vi "Estimate2DAffineVariableScale.vi"(8 "error in":errorcluster, 10 "To":map{i32, T1}(c390), 11 "From":map{i32, T1}(c390)) -> (0 "error out":errorcluster, 1 "c":dbl, 2 "T":T1, 3 "R":T2)   [LabVIEW 2020, in "ar.lvlib"]
doc: "Estimate an Affine Transformation between sets of points."
uses:
  ar.lvlib
  common/Image Point (Float).ctl
  <vilib>/Analysis/Matrix/Datatypes/RealMatrix.ctl
  1dd33249-2402-4cc2-9784-1d2efc93c5c7.vi
  SubtractMeanFromPoints.vi
  CovarianceofPointSetsA&B.vi
  DecomposeCovarianceOfPointSetsA&B.vi
  <vilib>/Analysis/baseanly.llb/A x Vector.vi
  <vilib>/Analysis/baseanly.llb/Mean.vi
  <vilib>/Analysis/baseanly.llb/Mean (DBL).vi
  <vilib>/Analysis/baseanly.llb/A x B.vi
  <vilib>/Analysis/baseanly.llb/Real A x B.vi
  <vilib>/Analysis/baseanly.llb/Determinant.vi
  <vilib>/Analysis/baseanly.llb/Real Determinant.vi
  SVDForPointSetCovarainces.vi
  <vilib>/Analysis/_algsub.llb/Matrix Rank.vi
  <vilib>/Analysis/_algsub.llb/Real Matrix Rank.vi
  <vilib>/Analysis/_algsub.llb/Trace.vi
  <vilib>/Analysis/_algsub.llb/Real Matrix Trace.vi
  <vilib>/Utility/error.llb/Error Cluster From Error Code.vi
  <vilib>/Analysis/Matrix/Numeric/Conversions/Array To Matrix - RA2.vi
  <vilib>/Analysis/7linalg.llb/SVD Decomposition.vi
  <vilib>/Analysis/7linalg.llb/Real SVD Decomposition.vi
  <vilib>/Analysis/7linalg.llb/Create Special Matrix.vi
  <vilib>/Analysis/7linalg.llb/Create Special Real Matrix.vi
  <vilib>/Analysis/Matrix/Numeric/Multiply/Multiply - RM,R.vi
  common/common.lvlib
  <vilib>/Analysis/Matrix/NI_Matrix.lvlib
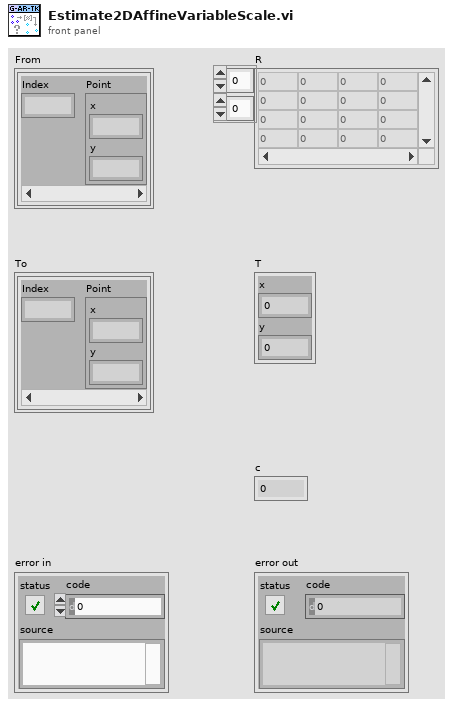
[diagram p1: front panel]
types:
  T1 = typedef "common.lvlib/Image Point (Float).ctl" = cluster{"x":dbl, "y":dbl}
  T2 = typedef "NI_Matrix.lvlib/RealMatrix.ctl" = dbl[][]
  T3 = typedef "ar.lvlib/PointSet.ctl" = dbl[][]
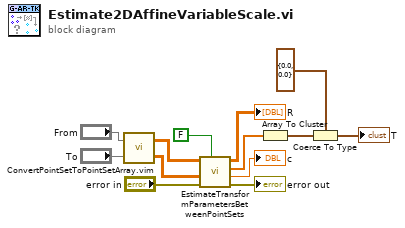
[diagram p0: block diagram]
diagram:
  n1 = call "ConvertPointSetToPointSetArray.vim"("To"="To", "From"="From") -> ("To Point Set"=w5:T3, "From Point Set"=w4:T3)
  n2 = call "EstimateTransformParametersBetweenPointSets.vi"("Fix Scale at 1.0?"=FALSE ("Fix Scale at 1.0"), "error in"="error in", "To Point Set"=w5, "From Point Set"=w4) -> ("error out"=→"error out":errorcluster, "c"=→"c":dbl, "t"=w1:dbl[], "R"=→"R":T2)  [unwired: 3 in, 1 out]
  n3 = Array To Cluster(array=w1) -> (cluster=w3:cluster{"t[0]":dbl, "t[1]":dbl})
  n4 = Coerce To Type(0:w3, 1:T1 {"x"=0.0, "y"=0.0} ("Image Point")) -> (2:→"T":T1)
